vi "_skipCPPStyleComment.vi"(8 "error in (no error)":errorcluster, 11 "JSON Parser In":refnum<class "tJSONParser.lvclass">) -> (0 "error out":errorcluster, 3 "JSON Parser Out":refnum<class "tJSONParser.lvclass">)   [LabVIEW 2013, in "JSON.lvlib" / "tJSONParser.lvclass"]
doc: "Consumes CPP-Style (//...) comments. Everything from \"//\" to the end of the line will be consumed and ignored for purposes of creating the JSON tree."
uses:
  tJSONParser.lvclass
  _tokenType.ctl
  tJSONParser.lvclass/tJSONParser.ctl
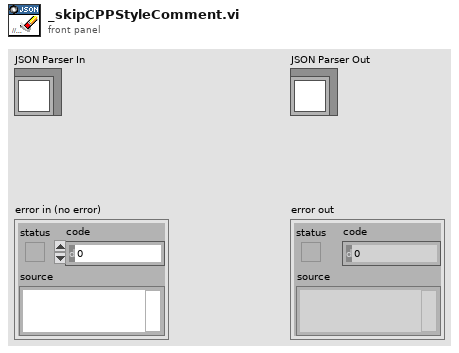
[diagram p1: front panel]
types:
  T1 = typedef "JSON.lvlib/tJSONParser.lvclass/_tokenType.ctl" = enum16{"Object Begin", "Object End", "Array Begin", "Array End", "String Delimeter", "Forward Slash", "Number", "Boolean", "Null", "Object Or Array Separator", "Pair Separator", "End Of File", "Asterisk", "Backward Slash", "Other"}
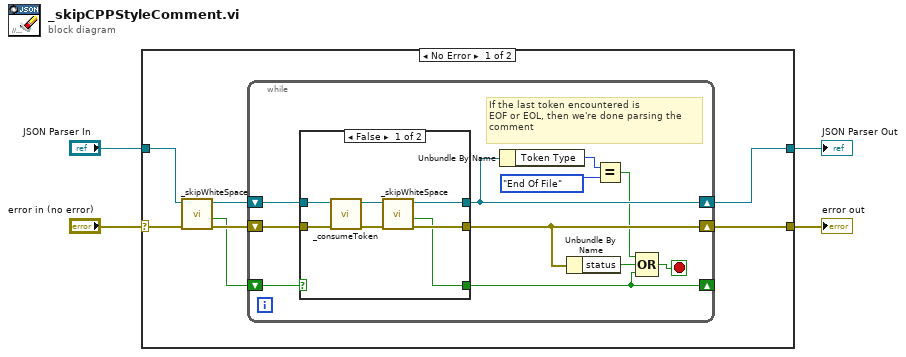
[diagram p0: block diagram]
diagram:
  n1 = case shown="No Error" "error in (no error)" {
    selector: "error in (no error)" -> [w11 w33]
    tunnel: [w8 w33] -> w3
    tunnel: "JSON Parser In" -> [w10 w34]
    tunnel: [w6 w34] -> w1
    frame No Error {
      n2 = call "_skipWhiteSpace.vi"("error in (no error)"=w11, "JSON Parser In"=w10) -> ("error out"=w9:errorcluster, "EOL Found?"=w5:bool, "JSON Parser Out"=w7:refnum<class "tJSONParser.lvclass">)  [unwired: 5 in, 2 out]
      n3 = while {
        shift-right: [w20] -> w8
        shift-left: w9 -> [w22]
        shift-right: [w15] -> w6
        shift-left: w7 -> [w21]
        shift-right: [w16] -> _
        shift-left: w5 -> [w17]
        stop <- w18 stop-if-true
        # "If the last token encountered is\nEOF or EOL, then we're done parsing the\ncomment"
        n4 = case shown="False" w17 {
          selector: w17 -> [_ w30]
          tunnel: w22 -> [w29 w31]
          tunnel: w21 -> [w28 w32]
          tunnel: [w25 w31] -> w20
          tunnel: [w23 w32] -> w15
          tunnel: [w24 w30] -> w16
          frame False {
            n5 = call "_consumeToken.vi"("error in (no error)"=w29, "JSON Parser In"=w28) -> ("error out"=w27:errorcluster, "JSON Parser Out"=w26:refnum<class "tJSONParser.lvclass">)  [unwired: 8 in]
            n6 = call "_skipWhiteSpace.vi"("error in (no error)"=w27, "JSON Parser In"=w26) -> ("error out"=w25:errorcluster, "EOL Found?"=w24:bool, "JSON Parser Out"=w23:refnum<class "tJSONParser.lvclass">)  [unwired: 5 in, 2 out]
          }
          frame True {
          }
        }
        n7 = Unbundle By Name(w15) -> ("Token Type"=w14:T1)
        n8 = Unbundle By Name(w20) -> ("status"=w19:bool)
        n9 = Equal?(x=w14, y=_tokenType."End Of File") -> (x = y?=w12:bool)
        n10 = Compound Arithmetic op=OR(w12, w19, w16) -> (w18:bool)
      }
    }
    frame Error {
    }
  }
  "error out" <- w3
  "JSON Parser Out" <- w1
